vi "ROS_Topic_Init.vi"(2 "node":string, 3 "Definitions":T1={"Topic"="/robot/head/command_head_nod", "Type"="std_msgs/Bool", "Action"=enum."Publisher", "Update (ms)"=1, "queue size"=1}) -> (0 "error out":errorcluster, 1 "ROS out":T3={"topic port"=0, "Node"="", "topic"="", "type"="", "node port"=0, "error "={"status"=FALSE, "code"=0, "source"=""}, "Direction"=enum."Node", "Update (ms)"=1, "queue size"=1})   [LabVIEW 2012]
doc: "Initializes a topic and returns a ROS cluster. Required before any read or write call."
uses:
  <userlib>/ROSforLV/ROS/Code/SubVIs/_ROSControl.ctl
  <userlib>/ROSforLV/ROS/Code/SubVIs/_ROSDirection.ctl
  <userlib>/ROSforLV/ROS/Code/Console/Servers/ServerSubs/TopicDef.ctl
  <userlib>/ROSforLV/ROS/Code/_ROSDefinition.vi
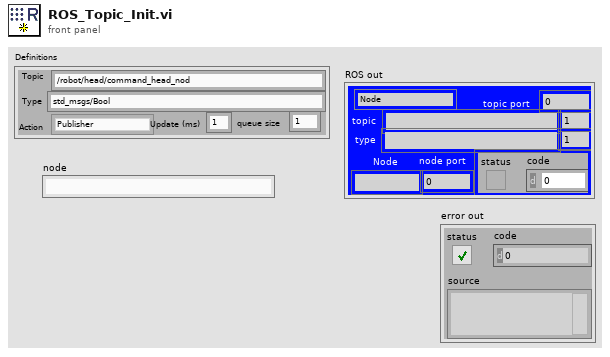
[diagram p1: front panel]
types:
  T1 = typedef "TopicDef.ctl" = cluster{"Topic":string, "Type":string, "Action":T2, "Update (ms)":u16, "queue size":u16}
  T2 = typedef "_ROSDirection.ctl" = enum16{"Node", "Publisher", "Subscriber", "Service Client"}
  T3 = typedef "_ROSControl.ctl" = cluster{"topic port":u16, "Node":string, "topic":string, "type":string, "node port":u16, "error ":errorcluster, "Direction":T2, "Update (ms)":u16, "queue size":u16}
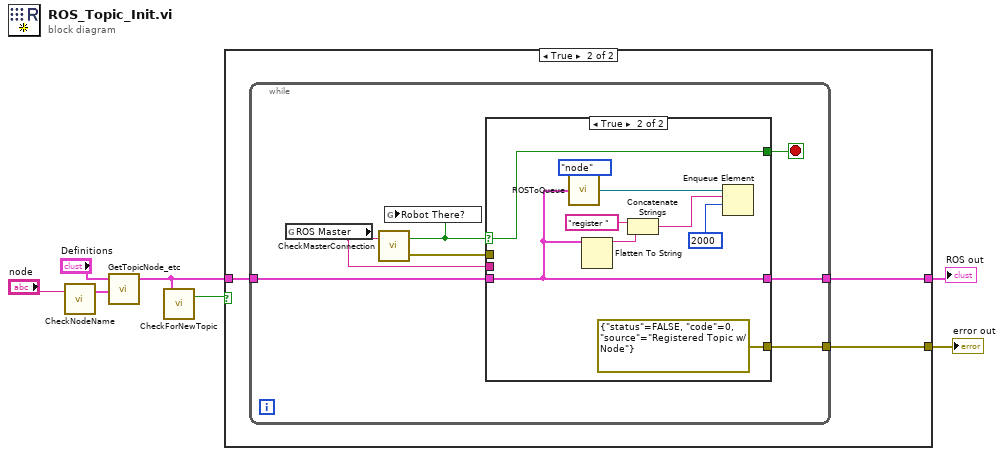
[diagram p0: block diagram]
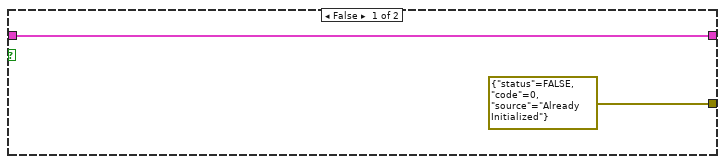
[diagram p2: hidden frame]
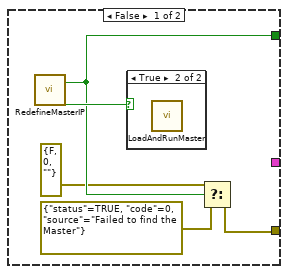
[diagram p3: hidden frame]
diagram:
  n1 = call <userlib>:"CheckNodeName.vi"("node"="node") -> ("Node"=w5:cluster{"name":string, "Port":u16})  [unwired: 1 in, 1 out]
  n2 = call <userlib>:"GetTopicNode_etc.vi"("Node"=w5, "Definitions"="Definitions") -> ("ROS"=w4:T3)  [unwired: 3 in]
  n3 = call <userlib>:"CheckForNewTopic.vi"("ROS"=w4) -> ("new?"=w3:bool)  [unwired: 2 in]
  n4 = case shown="True" w3 {
    tunnel: w4 -> [w9 w12]
    tunnel: [w9 w11] -> w6
    tunnel: [errorcluster {"status"=FALSE, "code"=0, "source"="Already Initialized"} ("error out") w10] -> w1
    frame False {
    }
    frame True {
      n5 = while {
        tunnel: w12 -> [w19]
        tunnel: [w15] -> w11
        tunnel: [w13] -> w10
        stop <- w14 stop-if-true
        n6 = global read "_ROSDefinition.vi" "ROS Master"() -> (w18:string)
        n7 = call <userlib>:"CheckMasterConnection.vi"("Master IP"=w18) -> ("error out"=w17:errorcluster, "Master There?"=w16:bool)  [unwired: 1 in]
        n8 = global write "_ROSDefinition.vi" "Robot There?"(w16) -> ()
        n9 = case shown="True" w16 {
          selector: w16 -> [_ w26]
          tunnel: w19 -> [_ w33]
          tunnel: [_ w33] -> w15
          tunnel: w18 -> [_ _]
          tunnel: w17 -> [_ _]
          tunnel: [w23 w26] -> w14
          tunnel: [w20 errorcluster {"status"=FALSE, "code"=0, "source"="Registered Topic w/ Node"} ("error out")] -> w13
          frame False {
            n10 = call <userlib>:"RedefineMasterIP.vi"() -> ("Abort?"=w23:bool, "Start Master"=w24:bool)  [unwired: 1 in]
            n11 = case shown="True" w24 {
              frame False {
              }
              frame True {
                n12 = call <userlib>:"LoadAndRunMaster.vi"() -> ()  [unwired: 2 in, 2 out]
              }
            }
            n13 = Select(t=errorcluster {"status"=FALSE, "code"=0, "source"=""} ("error out"), s=w23, f=errorcluster {"status"=TRUE, "code"=0, "source"="Failed to find the Master"} ("error out")) -> (s? t:f=w20:errorcluster)
          }
          frame True {
            n14 = call <userlib>:"ROSToQueue.vi"("ROS"=w33, "Name"=enum16{"topic", "node"}."node") -> ("queue"=w29:refnum<queue>)  [unwired: 2 in, 1 out]
            n15 = Flatten To String(anything=w33) -> (data string=w32:string)  [unwired: 3 in, 2 out]
            n16 = Concatenate Strings("register " ("string"), w32) -> (w31:string)
            n17 = Enqueue Element(queue=w29, element=w31, timeout in ms (-1)=2000) -> ()  [unwired: 1 in, 3 out]
          }
        }
      }
    }
  }
  "ROS out" <- w6
  "error out" <- w1
